vi "Autonomous Independent.vi"() -> ()   [LabVIEW 2018]
doc: "This VI is called when autonomous begins, and will automatically be terminated when autonomous ends. You can carry out timed or sensor driven robot movement independently without needing to return to the caller."
uses:
  <vilib>/Rock Robotics/WPI/Solenoid/WPI_SolenoidValue.ctl
  <vilib>/Rock Robotics/WPI/ThirdParty/Phoenix-LabVIEW/Motor Controller/Controls/CTRE_Phoenix_MotorControl_ControlMode.ctl
  <vilib>/Rock Robotics/WPI/Utilities/WPI_GetSetVariantRefNum.vi
  <vilib>/Rock Robotics/Network Tables/NT Write Numeric Array.vi
  <vilib>/Rock Robotics/WPI/Solenoid/WPI_SolenoidSetEnum.vi
  <vilib>/Rock Robotics/WPI/RobotDrive/WPI_RobotDriveArcadeDrive_Standard(NoSaturation).vi
  <vilib>/Rock Robotics/Network Tables/NT Read String.vi
  <vilib>/Rock Robotics/Network Tables/NT Write Boolean Array.vi
  <vilib>/Rock Robotics/Network Tables/NT Read Number.vi
panel:
  in  "Butterfly Status":bool=TRUE
  in  "ScoreMode":T1(ring)
  out "Current Movement, for debugging":T2 {"Y Joystick Value" scale=1.0..-1.0; "X Joystick Value" scale=-1.0..1.0}
  in  "Array of robot movements":T3(array[cluster])=[{"X Joystick Value"=0.39393939393939403, "Y Joystick Value"=0.0, "Delay (sec)"=1.0, "Movement Name"="turn"}, {"X Joystick Value"=-0.3737373737373737, "Y Joystick Value"=0.0, "Delay (sec)"=1.0, "Movement Name"="turn back"}] {"Y Joystick Value" scale=1.0..-1.0; "X Joystick Value" scale=-1.0..1.0}
  # "Be sure to right-click and choose Data Operations>>Make Current Value default if you want to save the array values with the VI"
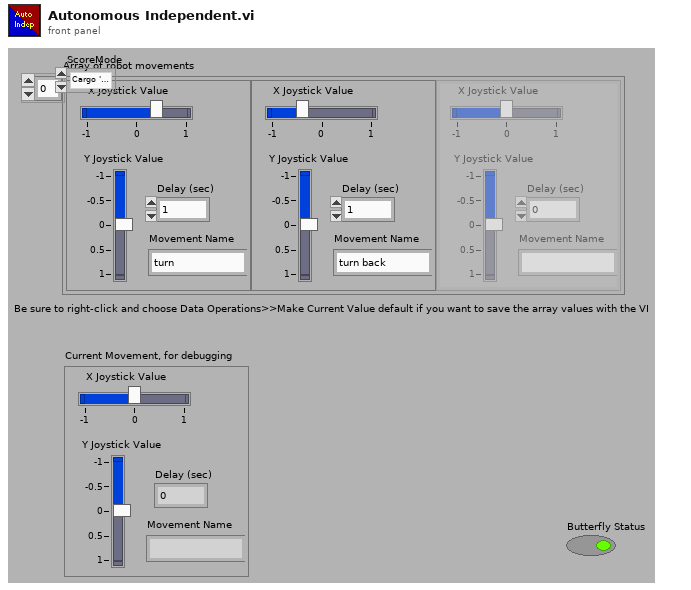
[diagram p1: front panel]
types:
  T1 = enum16{"Cargo 'default'", "Hatch", "HorseDriveHatch"}
  T2 = cluster{"X Joystick Value":dbl, "Y Joystick Value":dbl, "Delay (sec)":dbl, "Movement Name":string}
  T3 = cluster{"X Joystick Value":dbl, "Y Joystick Value":dbl, "Delay (sec)":dbl, "Movement Name":string}[]
  T4 = typedef "WPI_JoystickDevRef.ctl" = cluster{"Device":T5}
  T5 = typedef "WPI_JoystickDeviceEnum.ctl" = enum16{"USB 0", "USB 1", "USB 2", "USB 3", "USB 4", "USB 5"}
  T6 = typedef "WPI_SolenoidValue.ctl" = enum16{"Off", "On", "Forward", "Reverse"}
  T7 = typedef "CTRE_Phoenix_MotorControl_ControlMode.ctl" = u16
  T8 = typedef "WPI_MotorControlDeviceRef.ctl" = cluster{"DeviceStatus":errorcluster, "Type":T9, "PWM":cluster{"PWM Channel":T10, "DeadBand":T11}, "CAN":cluster{"Device Number":u8, "SetOutput VI Ref":variant, "GetOutput VI Ref":variant, "Enable VI Ref":variant, "Disable VI Ref":variant, "Data":variant}, "Invert":bool, "DIO PWM":cluster{"PWM \"Enable\" Channel":T10, "DIOChannel":T12, "PWM Rate":dbl}}
  T9 = typedef "WPI_MotorControlType.ctl" = enum16{"PWM", "CAN", "DIO PWM"}
  T10 = typedef "FPGA_DIOPWMChannel.ctl" = enum8{"PWM 0", "PWM 1", "PWM 2", "PWM 3", "PWM 4", "PWM 5", "PWM 6", "PWM 7", "PWM 8", "PWM 9", "PWM MXP 0", "PWM MXP 1", "PWM MXP 2", "PWM MXP 3", "PWM MXP 4", "PWM MXP 5", "PWM MXP 6", "PWM MXP 7", "PWM MXP 8", "PWM MXP 9", "Invalid"}
  T11 = typedef "WPI_PWMDeadband.ctl" = cluster{"Name":string, "maxPositivePwm":i32, "minPositivePwm":i32, "centerPwm":i32, "maxNegativePwm":i32, "minNegativePwm":i32, "angularRange":u16}
  T12 = typedef "FPGA_DIOChannel.ctl" = enum8{"DIO 0", "DIO 1", "DIO 2", "DIO 3", "DIO 4", "DIO 5", "DIO 6", "DIO 7", "DIO 8", "DIO 9", "DIO MXP 0", "DIO MXP 1", "DIO MXP 2", "DIO MXP 3", "DIO MXP 4", "DIO MXP 5", "DIO MXP 6", "DIO MXP 7", "DIO MXP 8", "DIO MXP 9", "DIO MXP 10", "DIO MXP 11", "DIO MXP 12", "DIO MXP 13", "DIO MXP 14", "DIO MXP 15", "SPI Port CS1", "SPI Port CS2", "SPI Port CS3", "SPI Port MISO", "SPI Port MOSI", "Invalid"}
  T13 = typedef "WPI_SolenoidDevRef.ctl" = cluster{"DevStatus":errorcluster, "Pneumatics Control Module":u8, "Forward Solenoid Channel":T14, "Reverse Solenoid Channel":T14}
  T14 = typedef "WPI_SolenoidChannel.ctl" = enum8{"Solenoid 0", "Solenoid 1", "Solenoid 2", "Solenoid 3", "Solenoid 4", "Solenoid 5", "Solenoid 6", "Solenoid 7", "Invalid"}
  T15 = typedef "WPI_RobotDriveDevRef.ctl" = cluster{"DevStatus":errorcluster, "Motors[]":T8[], "Square Inputs":bool, "Max Output":dbl}
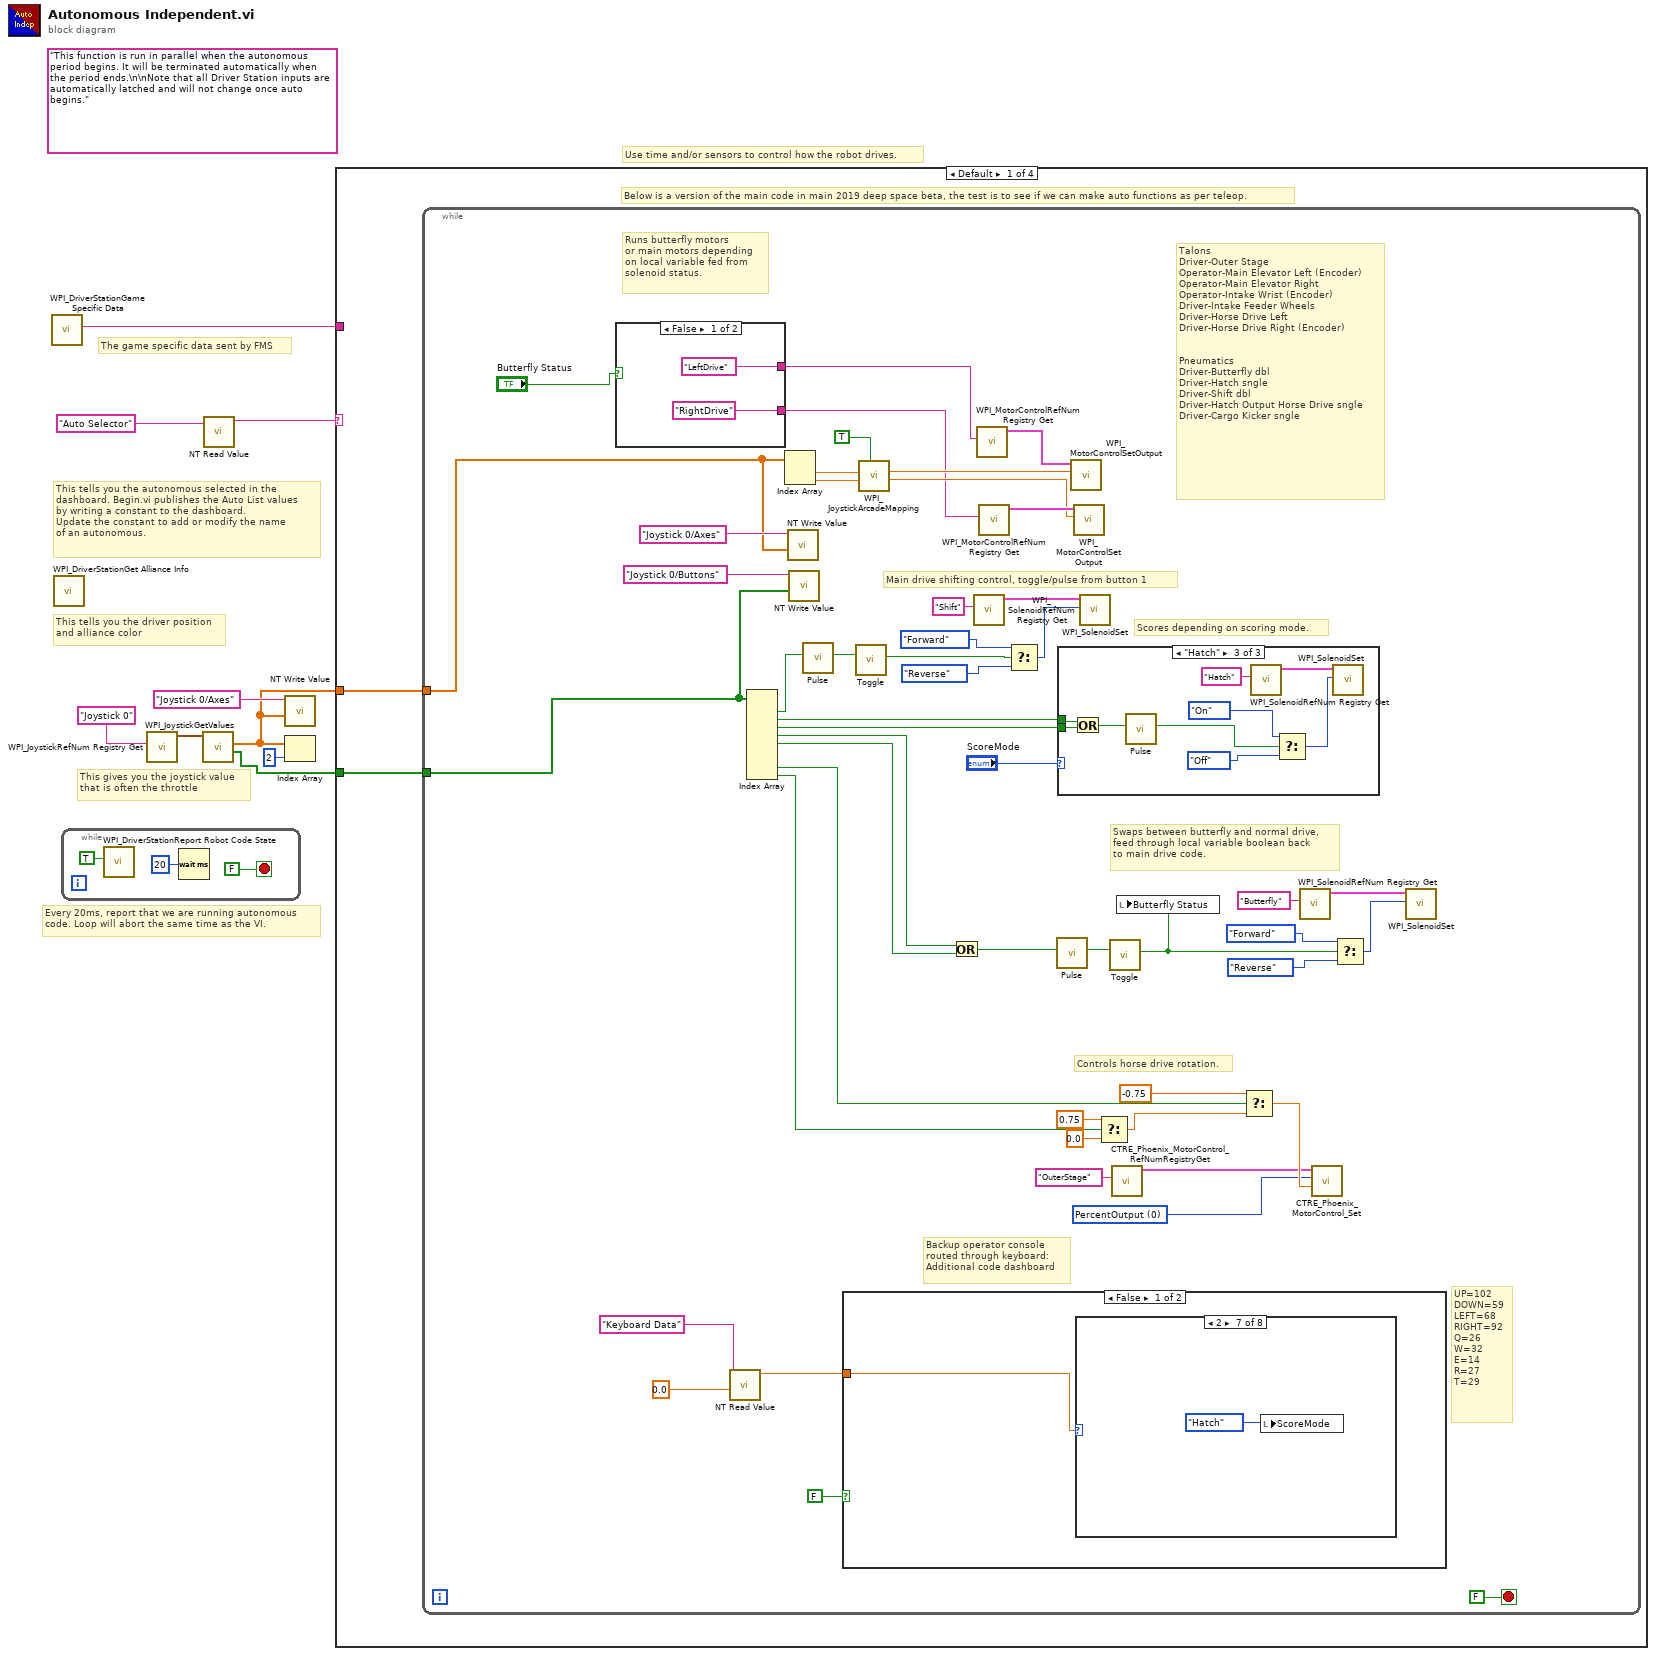
[diagram p0: block diagram]
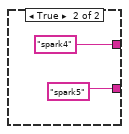
[diagram p2: hidden frame]
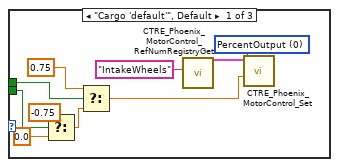
[diagram p3: hidden frame]
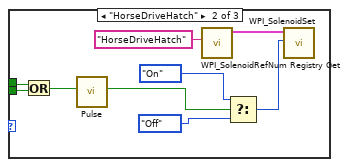
[diagram p4: hidden frame]
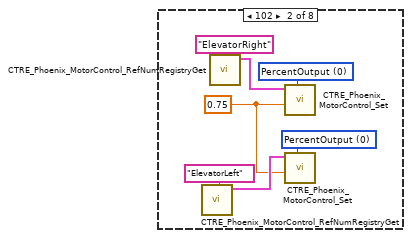
[diagram p6: hidden frame]
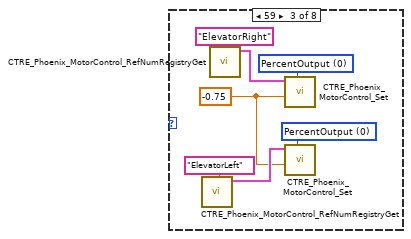
[diagram p7: hidden frame]
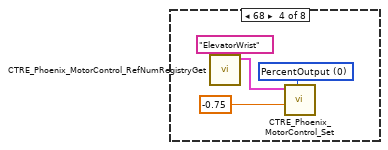
[diagram p8: hidden frame]
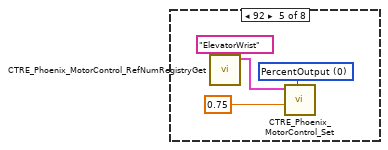
[diagram p9: hidden frame]
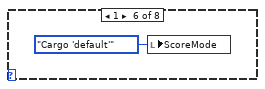
[diagram p10: hidden frame]
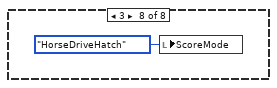
[diagram p11: hidden frame]
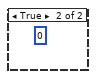
[diagram p12: hidden frame]
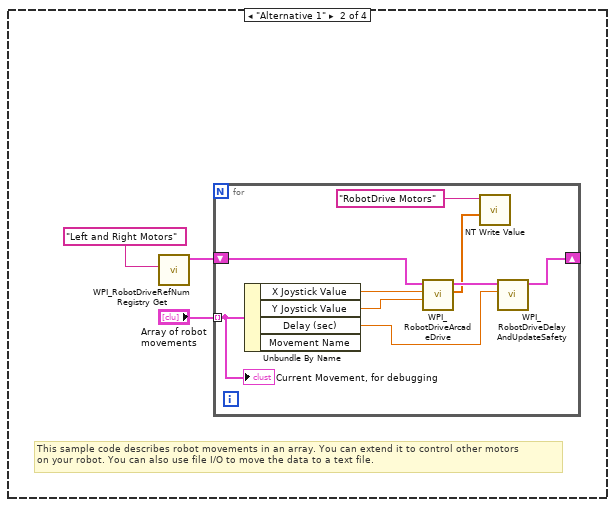
[diagram p13: hidden frame]
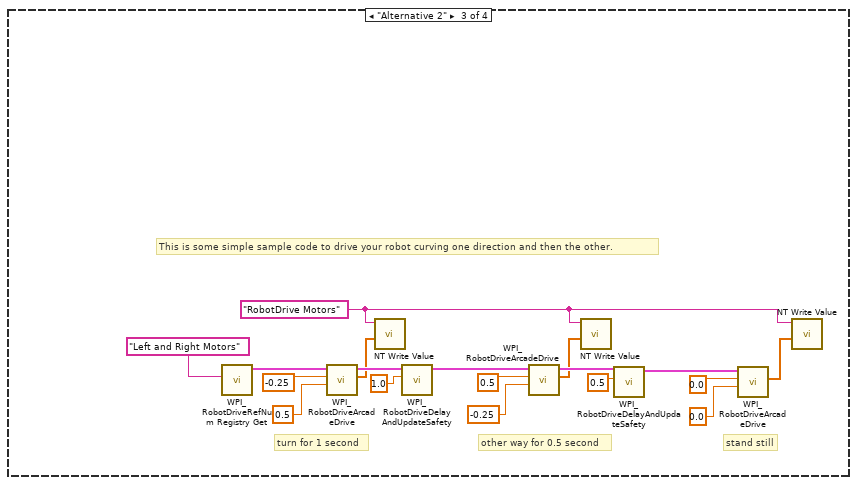
[diagram p14: hidden frame]
diagram:
  (unwired) "This function is run in parallel when the autonomous period begins. It will be terminated automatically when the period ends.\n\nNote that all Driver Station inputs are automatically latched and will not change once auto begins."
  # "The game specific data sent by FMS"
  # "This tells you the autonomous selected in the \ndashboard. Begin.vi publishes the Auto List values\nby writing a constant to the dashboard.\nUpdate the constant to add or modify the name\nof an autonomous."
  # "Every 20ms, report that we are running autonomous\ncode. Loop will abort the same time as the VI."
  # "This gives you the joystick value\nthat is often the throttle"
  # "Use time and/or sensors to control how the robot drives."
  # "This tells you the driver position\nand alliance color"
  n1 = call <vilib>:"WPI_DriverStationGame Specific Data.vi"() -> ("Game Specific Data"=w3:string)  [unwired: 11 in]
  n2 = call <vilib>:"WPI_DriverStationGet Alliance Info.vi"() -> ()  [unwired: 12 out]
  n3 = while {
    stop <- FALSE stop-if-true
    n4 = call <vilib>:"WPI_DriverStationReport Robot Code State.vi"("Autonomous"=TRUE) -> ()  [unwired: 10 in, 1 out]
    n5 = Wait (ms)(milliseconds to wait=u32 20) -> ()  [unwired: 1 out]
  }
  n6 = call <vilib>:"WPI_JoystickRefNum Registry Get.vi"("refnum name"="Joystick 0") -> ("JoystickDevRef"=w8:T4)  [unwired: 1 in, 9 out]
  n7 = call <vilib>:"WPI_JoystickGetValues.vi"("JoystickDevRef"=w8) -> ("Buttons"=w1:bool[], "Axes"=w2:dbl[])  [unwired: 6 in, 3 out]
  n8 = call-poly <vilib>:"NT Read Value.vi"("Name"="Auto Selector") -> ("String"=w5:string)  [unwired: 9 in, 1 out]
  n9 = call-poly <vilib>:"NT Write Value.vi"("Numeric Array"=w2, "Name"="Joystick 0/Axes") -> ()  [unwired: 9 in, 1 out]
  n10 = Index Array(array=w2, index=2) -> ()  [unwired: 1 out]
  n11 = case shown="Default" w5 {
    tunnel: w3 -> [_ _ _ _]
    tunnel: w2 -> [w14 _ _ _]
    tunnel: w1 -> [w13 _ _ _]
    frame Default {
      # "Below is a version of the main code in main 2019 deep space beta, the test is to see if we can make auto functions as per teleop."
      n12 = while {
        tunnel: w14 -> [w31]
        tunnel: w13 -> [w30]
        stop <- FALSE stop-if-true
        w27 = T7 0 items=["PercentOutput"=0, "Position"=1, "Velocity"=2, "Current"=3, "Follower"=5, "MotionProfile"=6, "MotionMagic"=7, "MotionProfileArc"=10, "Disabled"=15] ("Control Mode")
        # "UP=102\nDOWN=59\nLEFT=68\nRIGHT=92\nQ=26\nW=32\nE=14\nR=27\nT=29"
        # "Backup operator console\nrouted through keyboard:\nAdditional code dashboard"
        # "Controls horse drive rotation."
        # "Swaps between butterfly and normal drive,\nfeed through local variable boolean back\nto main drive code."
        # "Scores depending on scoring mode."
        # "Main drive shifting control, toggle/pulse from button 1"
        # "Runs butterfly motors\nor main motors depending\non local variable fed from\nsolenoid status."
        # "Talons\nDriver-Outer Stage \nOperator-Main Elevator Left (Encoder)\nOperator-Main Elevator Right\nOperator-Intake Wrist (Encoder)\nDriver-Intake Feeder Wheels\nDriver-Horse Drive Left\nDriver-Horse Drive Right (Encoder)\n\n\nPneumatics\nDriver-Butterfly dbl \nDriver-Hatch sngle\nDriver-Shift dbl\nDriver-Hatch Output Horse Drive sngle\nDriver-Cargo Kicker sngle"
        n13 = case shown="False" "Butterfly Status" {
          tunnel: ["LeftDrive" ("refnum name") "spark4" ("refnum name")] -> w17
          tunnel: ["RightDrive" ("refnum name") "spark5" ("refnum name")] -> w16
          frame False {
          }
          frame True {
          }
        }
        n14 = call-poly <vilib>:"NT Read Value.vi"("Default Value"=0.0, "Name"="Keyboard Data") -> ("Numeric"=w32:dbl)  [unwired: 8 in, 1 out]
        n15 = Index Array(array=w30) -> (element #1=w51:bool, element #2=w47:bool, element #3=w46:bool, element #4=w43:bool, element #5=w42:bool, element #8=w20:bool, element #9=w19:bool)  [unwired: 9 in, 2 out]
        n16 = Index Array(array=w31) -> (element #1=w62:dbl, element #2=w61:dbl)  [unwired: 2 in]
        n17 = call-poly <vilib>:"NT Write Value.vi"("Numeric Array"=w31, "Name"="Joystick 0/Axes") -> ()  [unwired: 9 in, 1 out]
        n18 = call-poly <vilib>:"NT Write Value.vi"("Boolean Array"=w30, "Name"="Joystick 0/Buttons") -> ()  [unwired: 9 in, 1 out]
        n19 = call "Pulse.vi"("Input"=w51) -> ("Output"=w50:bool)  [unwired: 10 in]
        n20 = case shown="False" FALSE {
          tunnel: w32 -> [w97 _]
          frame False {
            n21 = case shown="2" w97 {
              frame 0, Default {
              }
              frame 102 {
                w98 = 0.75 ("Output")
                w100 = T7 0 items=["PercentOutput"=0, "Position"=1, "Velocity"=2, "Current"=3, "Follower"=5, "MotionProfile"=6, "MotionMagic"=7, "MotionProfileArc"=10, "Disabled"=15] ("Control Mode")
                w104 = T7 0 items=["PercentOutput"=0, "Position"=1, "Velocity"=2, "Current"=3, "Follower"=5, "MotionProfile"=6, "MotionMagic"=7, "MotionProfileArc"=10, "Disabled"=15] ("Control Mode")
                n22 = call <vilib>:"CTRE_Phoenix_MotorControl_RefNumRegistryGet.vi"("refnum name"="ElevatorLeft") -> ("PhoenixMotorControlDevRef"=w101:T8)  [unwired: 9 in, 1 out]
                n23 = call <vilib>:"CTRE_Phoenix_MotorControl_RefNumRegistryGet.vi"("refnum name"="ElevatorRight") -> ("PhoenixMotorControlDevRef"=w103:T8)  [unwired: 9 in, 1 out]
                n24 = call <vilib>:"CTRE_Phoenix_MotorControl_Set.vi"("Output"=w98, "Control Mode"=w104, "PhoenixMotorControlDevRef"=w103) -> ()  [unwired: 7 in, 2 out]
                n25 = call <vilib>:"CTRE_Phoenix_MotorControl_Set.vi"("Output"=w98, "Control Mode"=w100, "PhoenixMotorControlDevRef"=w101) -> ()  [unwired: 7 in, 2 out]
              }
              frame 59 {
                w105 = -0.75 ("Output")
                w107 = T7 0 items=["PercentOutput"=0, "Position"=1, "Velocity"=2, "Current"=3, "Follower"=5, "MotionProfile"=6, "MotionMagic"=7, "MotionProfileArc"=10, "Disabled"=15] ("Control Mode")
                w111 = T7 0 items=["PercentOutput"=0, "Position"=1, "Velocity"=2, "Current"=3, "Follower"=5, "MotionProfile"=6, "MotionMagic"=7, "MotionProfileArc"=10, "Disabled"=15] ("Control Mode")
                n26 = call <vilib>:"CTRE_Phoenix_MotorControl_RefNumRegistryGet.vi"("refnum name"="ElevatorLeft") -> ("PhoenixMotorControlDevRef"=w108:T8)  [unwired: 9 in, 1 out]
                n27 = call <vilib>:"CTRE_Phoenix_MotorControl_RefNumRegistryGet.vi"("refnum name"="ElevatorRight") -> ("PhoenixMotorControlDevRef"=w110:T8)  [unwired: 9 in, 1 out]
                n28 = call <vilib>:"CTRE_Phoenix_MotorControl_Set.vi"("Output"=w105, "Control Mode"=w111, "PhoenixMotorControlDevRef"=w110) -> ()  [unwired: 7 in, 2 out]
                n29 = call <vilib>:"CTRE_Phoenix_MotorControl_Set.vi"("Output"=w105, "Control Mode"=w107, "PhoenixMotorControlDevRef"=w108) -> ()  [unwired: 7 in, 2 out]
              }
              frame 68 {
                w115 = T7 0 items=["PercentOutput"=0, "Position"=1, "Velocity"=2, "Current"=3, "Follower"=5, "MotionProfile"=6, "MotionMagic"=7, "MotionProfileArc"=10, "Disabled"=15] ("Control Mode")
                n30 = call <vilib>:"CTRE_Phoenix_MotorControl_RefNumRegistryGet.vi"("refnum name"="ElevatorWrist") -> ("PhoenixMotorControlDevRef"=w114:T8)  [unwired: 9 in, 1 out]
                n31 = call <vilib>:"CTRE_Phoenix_MotorControl_Set.vi"("Output"=-0.75, "Control Mode"=w115, "PhoenixMotorControlDevRef"=w114) -> ()  [unwired: 7 in, 2 out]
              }
              frame 92 {
                w119 = T7 0 items=["PercentOutput"=0, "Position"=1, "Velocity"=2, "Current"=3, "Follower"=5, "MotionProfile"=6, "MotionMagic"=7, "MotionProfileArc"=10, "Disabled"=15] ("Control Mode")
                n32 = call <vilib>:"CTRE_Phoenix_MotorControl_RefNumRegistryGet.vi"("refnum name"="ElevatorWrist") -> ("PhoenixMotorControlDevRef"=w118:T8)  [unwired: 9 in, 1 out]
                n33 = call <vilib>:"CTRE_Phoenix_MotorControl_Set.vi"("Output"=0.75, "Control Mode"=w119, "PhoenixMotorControlDevRef"=w118) -> ()  [unwired: 7 in, 2 out]
              }
              frame 1 {
                n34 = local write "ScoreMode"(T1."Cargo 'default'" ("ScoreMode")) -> ()
              }
              frame 2 {
                n35 = local write "ScoreMode"(T1."Hatch" ("ScoreMode")) -> ()
              }
              frame 3 {
                n36 = local write "ScoreMode"(T1."HorseDriveHatch" ("ScoreMode")) -> ()
              }
            }
          }
          frame True {
            (unwired) 0
          }
        }
        n37 = call "Toggle.vi"("Input"=w50) -> ("Output"=w49:bool)  [unwired: 10 in]
        n38 = call <vilib>:"WPI_JoystickArcadeMapping.vi"("Square Inputs"=TRUE, "Y axis value"=w61, "X axis value"=w62) -> ("Right Motor Value"=w56:dbl, "Left Motor Value"=w58:dbl)  [unwired: 7 in]
        n39 = Or(x=w43, y=w42) -> (x .or. y?=w41:bool)
        n40 = call <vilib>:"WPI_SolenoidRefNum Registry Get.vi"("refnum name"="Shift") -> ("SolenoidDevRef"=w54:T13)  [unwired: 9 in, 1 out]
        n41 = call <vilib>:"WPI_MotorControlRefNum Registry Get.vi"("refnum name"=w17) -> ("MotorControlDevRef"=w59:T8)  [unwired: 9 in, 1 out]
        n42 = call <vilib>:"WPI_MotorControlRefNum Registry Get.vi"("refnum name"=w16) -> ("MotorControlDevRef"=w57:T8)  [unwired: 9 in, 1 out]
        n43 = Select(t=WPI_SolenoidValue."Forward" ("Value"), s=w49, f=WPI_SolenoidValue."Reverse" ("Value")) -> (s? t:f=w48:T6)
        n44 = call "Pulse.vi"("Input"=w41) -> ("Output"=w45:bool)  [unwired: 10 in]
        n45 = case shown="\"Hatch\"" "ScoreMode" {
          tunnel: w47 -> [w75 w84 w93]
          tunnel: w46 -> [w74 w85 w94]
          frame "Cargo 'default'", Default {
            w76 = T7 0 items=["PercentOutput"=0, "Position"=1, "Velocity"=2, "Current"=3, "Follower"=5, "MotionProfile"=6, "MotionMagic"=7, "MotionProfileArc"=10, "Disabled"=15] ("Control Mode")
            n46 = Select(t=-0.75, s=w74, f=0.0) -> (s? t:f=w73:dbl)
            n47 = Select(t=0.75, s=w75, f=w73) -> (s? t:f=w69:dbl)
            n48 = call <vilib>:"CTRE_Phoenix_MotorControl_RefNumRegistryGet.vi"("refnum name"="IntakeWheels") -> ("PhoenixMotorControlDevRef"=w77:T8)  [unwired: 9 in, 1 out]
            n49 = call <vilib>:"CTRE_Phoenix_MotorControl_Set.vi"("Output"=w69, "Control Mode"=w76, "PhoenixMotorControlDevRef"=w77) -> ()  [unwired: 7 in, 2 out]
          }
          frame "HorseDriveHatch" {
            n50 = Or(x=w84, y=w85) -> (x .or. y?=w83:bool)
            n51 = call "Pulse.vi"("Input"=w83) -> ("Output"=w82:bool)  [unwired: 10 in]
            n52 = call <vilib>:"WPI_SolenoidRefNum Registry Get.vi"("refnum name"="HorseDriveHatch") -> ("SolenoidDevRef"=w87:T13)  [unwired: 9 in, 1 out]
            n53 = Select(t=WPI_SolenoidValue."On" ("Value"), s=w82, f=WPI_SolenoidValue."Off" ("Value")) -> (s? t:f=w79:T6)
            n54 = call-poly <vilib>:"WPI_SolenoidSet.vi"("Value"=w79, "SolenoidDevRef"=w87) -> ()  [unwired: 8 in, 2 out]
          }
          frame "Hatch" {
            n55 = Or(x=w93, y=w94) -> (x .or. y?=w92:bool)
            n56 = call "Pulse.vi"("Input"=w92) -> ("Output"=w91:bool)  [unwired: 10 in]
            n57 = call <vilib>:"WPI_SolenoidRefNum Registry Get.vi"("refnum name"="Hatch") -> ("SolenoidDevRef"=w96:T13)  [unwired: 9 in, 1 out]
            n58 = Select(t=WPI_SolenoidValue."On" ("Value"), s=w91, f=WPI_SolenoidValue."Off" ("Value")) -> (s? t:f=w88:T6)
            n59 = call-poly <vilib>:"WPI_SolenoidSet.vi"("Value"=w88, "SolenoidDevRef"=w96) -> ()  [unwired: 8 in, 2 out]
          }
        }
        n60 = call <vilib>:"WPI_MotorControlSetOutput.vi"("Output"=w58, "MotorControlDevRef"=w59) -> ()  [unwired: 7 in, 3 out]
        n61 = call <vilib>:"WPI_MotorControlSetOutput.vi"("Output"=w56, "MotorControlDevRef"=w57) -> ()  [unwired: 7 in, 3 out]
        n62 = call-poly <vilib>:"WPI_SolenoidSet.vi"("Value"=w48, "SolenoidDevRef"=w54) -> ()  [unwired: 8 in, 2 out]
        n63 = Select(t=0.75, s=w19, f=0.0) -> (s? t:f=w21:dbl)
        n64 = call "Toggle.vi"("Input"=w45) -> ("Output"=w15:bool)  [unwired: 10 in]
        n65 = call <vilib>:"CTRE_Phoenix_MotorControl_RefNumRegistryGet.vi"("refnum name"="OuterStage") -> ("PhoenixMotorControlDevRef"=w26:T8)  [unwired: 9 in, 1 out]
        n66 = local write "Butterfly Status"(w15) -> ()
        n67 = Select(t=-0.75, s=w20, f=w21) -> (s? t:f=w28:dbl)
        n68 = call <vilib>:"WPI_SolenoidRefNum Registry Get.vi"("refnum name"="Butterfly") -> ("SolenoidDevRef"=w37:T13)  [unwired: 9 in, 1 out]
        n69 = call <vilib>:"CTRE_Phoenix_MotorControl_Set.vi"("Output"=w28, "Control Mode"=w27, "PhoenixMotorControlDevRef"=w26) -> ()  [unwired: 7 in, 2 out]
        n70 = Select(t=WPI_SolenoidValue."Forward" ("Value"), s=w15, f=WPI_SolenoidValue."Reverse" ("Value")) -> (s? t:f=w40:T6)
        n71 = call-poly <vilib>:"WPI_SolenoidSet.vi"("Value"=w40, "SolenoidDevRef"=w37) -> ()  [unwired: 8 in, 2 out]
      }
    }
    frame "Alternative 1" {
      # "This sample code describes robot movements in an array. You can extend it to control other motors\non your robot. You can also use file I/O to move the data to a text file."
      n72 = call <vilib>:"WPI_RobotDriveRefNum Registry Get.vi"("refnum name"="Left and Right Motors") -> ("RobotDriveDevRef"=w124:T15)  [unwired: 1 in, 9 out]
      n73 = for {
        shift-right: [w132] -> _
        shift-left: w124 -> [w133]
        tunnel: "Array of robot movements" -> [w128] mode=indexing
        n74 = Unbundle By Name(w128) -> ("X Joystick Value"=w131:dbl, "Y Joystick Value"=w130:dbl, "Delay (sec)"=w129:dbl)  [unwired: 1 out]
        n75 = call-poly <vilib>:"WPI_RobotDriveArcadeDrive.vi"("Y axis value"=w130, "X axis value"=w131, "RobotDriveDevRef"=w133) -> ("Motor Values"=w126:dbl[], "RobotDriveDevRef"=w134:T15)  [unwired: 1 in, 6 out]
        n76 = call-poly <vilib>:"NT Write Value.vi"("Numeric Array"=w126, "Name"="RobotDrive Motors") -> ()  [unwired: 9 in, 1 out]
        n77 = call <vilib>:"WPI_RobotDriveDelayAndUpdateSafety.vi"("Delay (s)"=w129, "RobotDriveDevRef"=w134) -> ("RobotDriveDevRef 2"=w132:T15)  [unwired: 8 in, 1 out]
        "Current Movement, for debugging" <- w128
      }
    }
    frame "Alternative 2" {
      w136 = "RobotDrive Motors" ("Name")
      # "This is some simple sample code to drive your robot curving one direction and then the other."
      # "stand still"
      # "other way for 0.5 second"
      # "turn for 1 second"
      n78 = call <vilib>:"WPI_RobotDriveRefNum Registry Get.vi"("refnum name"="Left and Right Motors") -> ("RobotDriveDevRef"=w152:T15)  [unwired: 1 in, 9 out]
      n79 = call-poly <vilib>:"WPI_RobotDriveArcadeDrive.vi"("Y axis value"=0.5 ("X axis value"), "X axis value"=-0.25, "RobotDriveDevRef"=w152) -> ("Motor Values"=w135:dbl[], "RobotDriveDevRef"=w145:T15)  [unwired: 1 in, 6 out]
      n80 = call-poly <vilib>:"NT Write Value.vi"("Numeric Array"=w135, "Name"=w136) -> ()  [unwired: 9 in, 1 out]
      n81 = call <vilib>:"WPI_RobotDriveDelayAndUpdateSafety.vi"("Delay (s)"=1.0, "RobotDriveDevRef"=w145) -> ("RobotDriveDevRef 2"=w146:T15)  [unwired: 8 in, 1 out]
      n82 = call-poly <vilib>:"WPI_RobotDriveArcadeDrive.vi"("Y axis value"=-0.25 ("X axis value"), "X axis value"=0.5, "RobotDriveDevRef"=w146) -> ("Motor Values"=w137:dbl[], "RobotDriveDevRef"=w147:T15)  [unwired: 1 in, 6 out]
      n83 = call-poly <vilib>:"NT Write Value.vi"("Numeric Array"=w137, "Name"=w136) -> ()  [unwired: 9 in, 1 out]
      n84 = call <vilib>:"WPI_RobotDriveDelayAndUpdateSafety.vi"("Delay (s)"=0.5, "RobotDriveDevRef"=w147) -> ("RobotDriveDevRef 2"=w148:T15)  [unwired: 8 in, 1 out]
      n85 = call-poly <vilib>:"WPI_RobotDriveArcadeDrive.vi"("Y axis value"=0.0 ("X axis value"), "X axis value"=0.0, "RobotDriveDevRef"=w148) -> ("Motor Values"=w138:dbl[])  [unwired: 1 in, 7 out]
      n86 = call-poly <vilib>:"NT Write Value.vi"("Numeric Array"=w138, "Name"=w136) -> ()  [unwired: 9 in, 1 out]
    }
    frame "Your Turn" {
    }
  }
